vi "Validate Client Names.vi"(8 "error in (no error)":errorcluster, 10 "project ref":refnum<vi>, 11 "multicolumnListbox in":refnum<vi>) -> (0 "error out":errorcluster, 2 "warning?":bool, 3 "multicolumnListbox out":refnum<vi>)   [LabVIEW 2021, in "Create Measurement Plug-In Client.lvlib"]
uses:
  Create Measurement Plug-In Client.lvlib
  <vilib>/Utility/miscctls.llb/LVRowAndColumnTypeDef.ctl
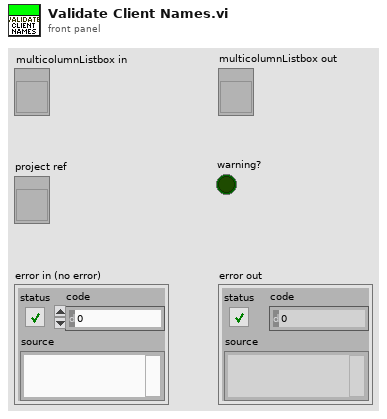
[diagram p1: front panel]
types:
  T1 = typedef "LVRowAndColumnTypeDef.ctl" = cluster{"Row":i32, "Column":i32}
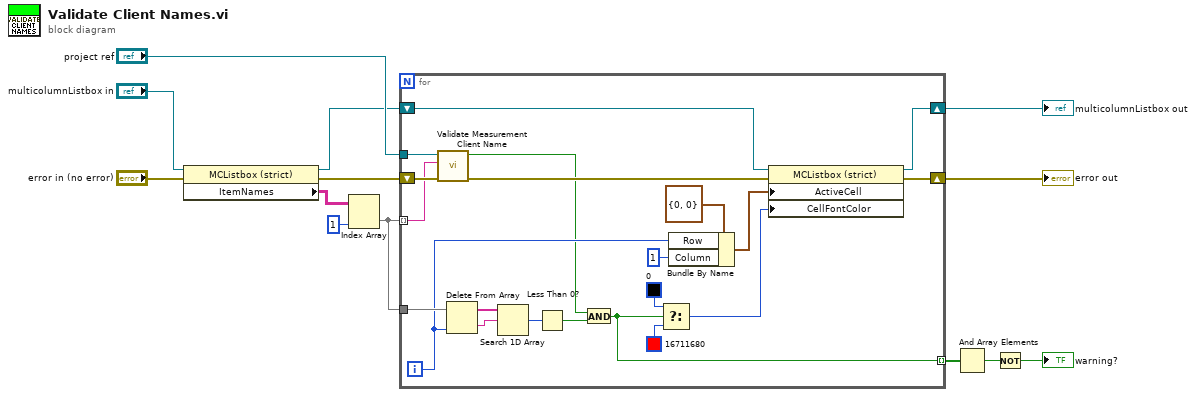
[diagram p0: block diagram]
diagram:
  n1 = property class="MCListbox (strict)"(reference="multicolumnListbox in", error in="error in (no error)") -> (reference out=w7:refnum<vi>, error out=w10:errorcluster, "ItemNames"=w13:string[][])
  n2 = Index Array(array=w13, index (col)=1 ("disabled index (col)")) -> (element=w2:string[])  [unwired: 1 in]
  n3 = for {
    shift-right: [w24] -> w6
    shift-left: w10 -> [w34]
    tunnel: w2 -> [w22] mode=indexing
    tunnel: "project ref" -> [w33]
    shift-right: [w23] -> w5
    shift-left: w7 -> [w31]
    tunnel: [w14] -> w4 mode=indexing
    tunnel: w2 -> [w21]
    i -> [w18]
    n4 = call "Validate Measurement Client Name.vi"("error in"=w34, "requested plugin name"=w22, "project ref"=w33) -> ("error out"=w32:errorcluster, "valid name?"=w15:bool)  [unwired: 7 in]
    n5 = Delete From Array(array=w21, index=w18) -> (deleted portion=w19:string, array with subset deleted=w20:string[])  [unwired: 1 in]
    n6 = Search 1D Array(1D array=w20, element=w19) -> (index of element=w17:i32)  [unwired: 1 in]
    n7 = Less Than 0?(x=w17) -> (x < 0?=w16:bool)
    n8 = And(x=w15, y=w16) -> (x .and. y?=w14:bool)
    n9 = Select(t=u32 0 ("Active Cell:Cell Font:Color"), s=w14, f=u32 16711680 ("Active Cell:Cell Font:Color")) -> (s? t:f=w25:u32)
    n10 = Bundle By Name(cluster=T1 {"Row"=0, "Column"=0} ("Active Cell:Active Cell"), "Row"=w18, "Column"=1) -> (w29:T1)
    n11 = property class="MCListbox (strict)"(reference=w31, error in=w32, "ActiveCell"=w29, "CellFontColor"=w25) -> (reference out=w23:refnum<vi>, error out=w24:errorcluster)
  }
  "error out" <- w6
  "multicolumnListbox out" <- w5
  n12 = And Array Elements(Boolean array=w4) -> (logical AND=w3:bool)
  n13 = Not(x=w3) -> (.not. x?=→"warning?":bool)
